vi "Transmit.vi"(8 "error in (no error)":errorcluster, 10 "log?":bool, 11 "Stream in":refnum<class "Stream.lvclass">) -> (0 "error out":errorcluster, 3 "Stream out":refnum<class "Stream.lvclass">)   [LabVIEW 2018, in "Stream.lvclass"]
uses:
  Stream.lvclass
  Stream.lvclass/Stream.ctl
  Comm.lvclass
panel:
  out "timed out?":bool
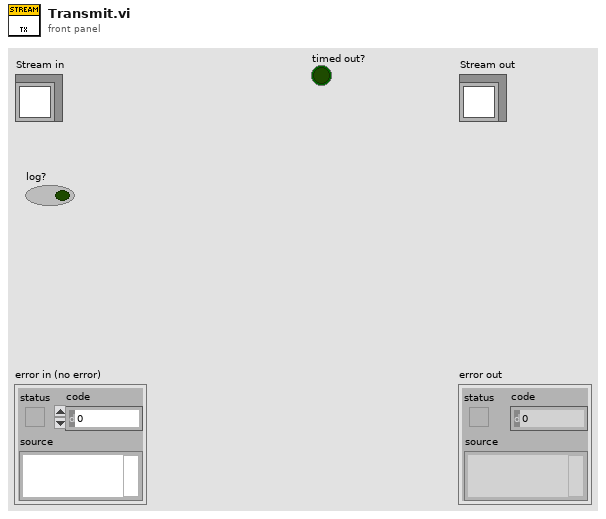
[diagram p1: front panel]
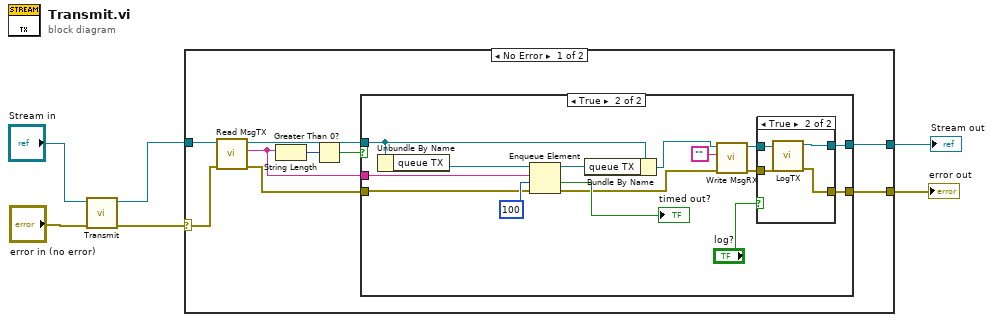
[diagram p0: block diagram]
diagram:
  n1 = call-parent "Transmit.vi"("error in (no error)"="error in (no error)", "Comm in"="Stream in") -> ("error out"=w4:errorcluster, "Comm out"=w3:refnum<class "Stream.lvclass">)  [unwired: 8 in]
  n2 = case shown="No Error" w4 {
    selector: w4 -> [w13 w39]
    tunnel: w3 -> [w15 w40]
    tunnel: [w11 w40] -> w2
    tunnel: [w10 w39] -> w1
    frame No Error {
      n3 = call-dynamic "Read MsgTX.vi"("error in (no error)"=w13, "Comm in"=w15) -> ("error out"=w9:errorcluster, "MsgTX"=w8:string, "Comm out"=w12:refnum<class "Stream.lvclass">)  [unwired: 7 in]
      n4 = String Length(string=w8) -> (length=w14:i32)
      n5 = Greater Than 0?(x=w14) -> (x > 0?=w7:bool)
      n6 = case shown="True" w7 {
        tunnel: w12 -> [w17 w31]
        tunnel: w8 -> [_ w32]
        tunnel: [w17 w27] -> w11
        tunnel: w9 -> [w16 w20]
        tunnel: [w16 w26] -> w10
        frame False {
        }
        frame True {
          n7 = Unbundle By Name(w31) -> ("queue TX"=w19:refnum<queue>)
          n8 = Enqueue Element(queue=w19, element=w32, timeout in ms (-1)=100, error in (no error)=w20) -> (queue out=w30:refnum<queue>, timed out?=→"timed out?":bool, error out=w25:errorcluster)
          n9 = Bundle By Name(cluster=w31, "queue TX"=w30) -> (w24:refnum<class "Stream.lvclass">)
          n10 = call-dynamic "Write MsgRX.vi"("error in (no error)"=w25, "MsgRX"="", "Comm in"=w24) -> ("error out"=w22:errorcluster, "Comm out"=w21:refnum<class "Stream.lvclass">)  [unwired: 7 in]
          n11 = case shown="True" "log?" {
            tunnel: [w34 w38] -> w27
            tunnel: [w33 w37] -> w26
            tunnel: w22 -> [w33 w36]
            tunnel: w21 -> [w34 w35]
            frame False {
            }
            frame True {
              n12 = call-dynamic "LogTX.vi"("error in (no error)"=w36, "Stream in"=w35) -> ("error out"=w37:errorcluster, "Stream out"=w38:refnum<class "Stream.lvclass">)  [unwired: 8 in]
            }
          }
        }
      }
    }
    frame Error {
    }
  }
  "error out" <- w1
  "Stream out" <- w2
